vi "Keithley2200series_2_ST.vi"() -> ()   [LabVIEW 2010]
uses:
  <vilib>/Utility/error.llb/whitespace.ctl
  C:/Users/rad/Desktop/Keithley 2200 Series Power Supplies Ver 1.2 (LV2009)/Keithley 2200 Series/Keithley 2200 Series.lvlib
panel:
  in  "ИС":string="5962-9683901MPA"
  in  "№ ИС":string
  out "SEE1 Count 2":dbl
  out "SEE1 Count":dbl
  in  "SEE th 2":dbl
  in  "SEE th 1":dbl
  in  "+ИП2":bool
  out "MEAS 2":string
  in  "Cml set 2":dbl
  in  "Function(0:Voltage) 3":u16(ring) items=["Voltage", "Current"]
  in  "Out set 2":dbl
  in  "VISA resource name 2":refnum<visa-resource-name>
  in  "Cml set":dbl
  in  "Function(0:Voltage) 2":u16(ring) items=["Voltage", "Current"]
  in  "Out set":dbl
  in  "Файл записи замеров":path
  out "MEAS":string
  in  "VISA resource name":refnum<visa-resource-name>
  in  "stop":bool
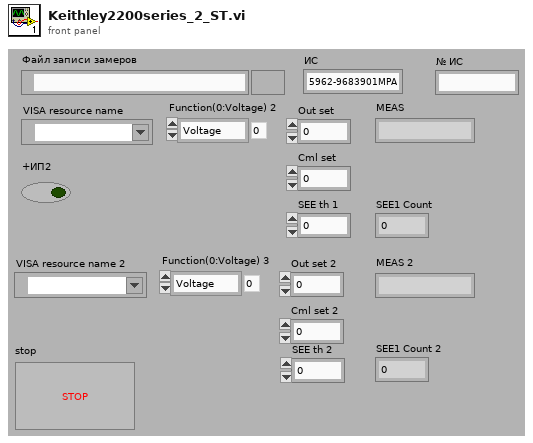
[diagram p1: front panel]
types:
  T1 = typedef "whitespace.ctl" = u16
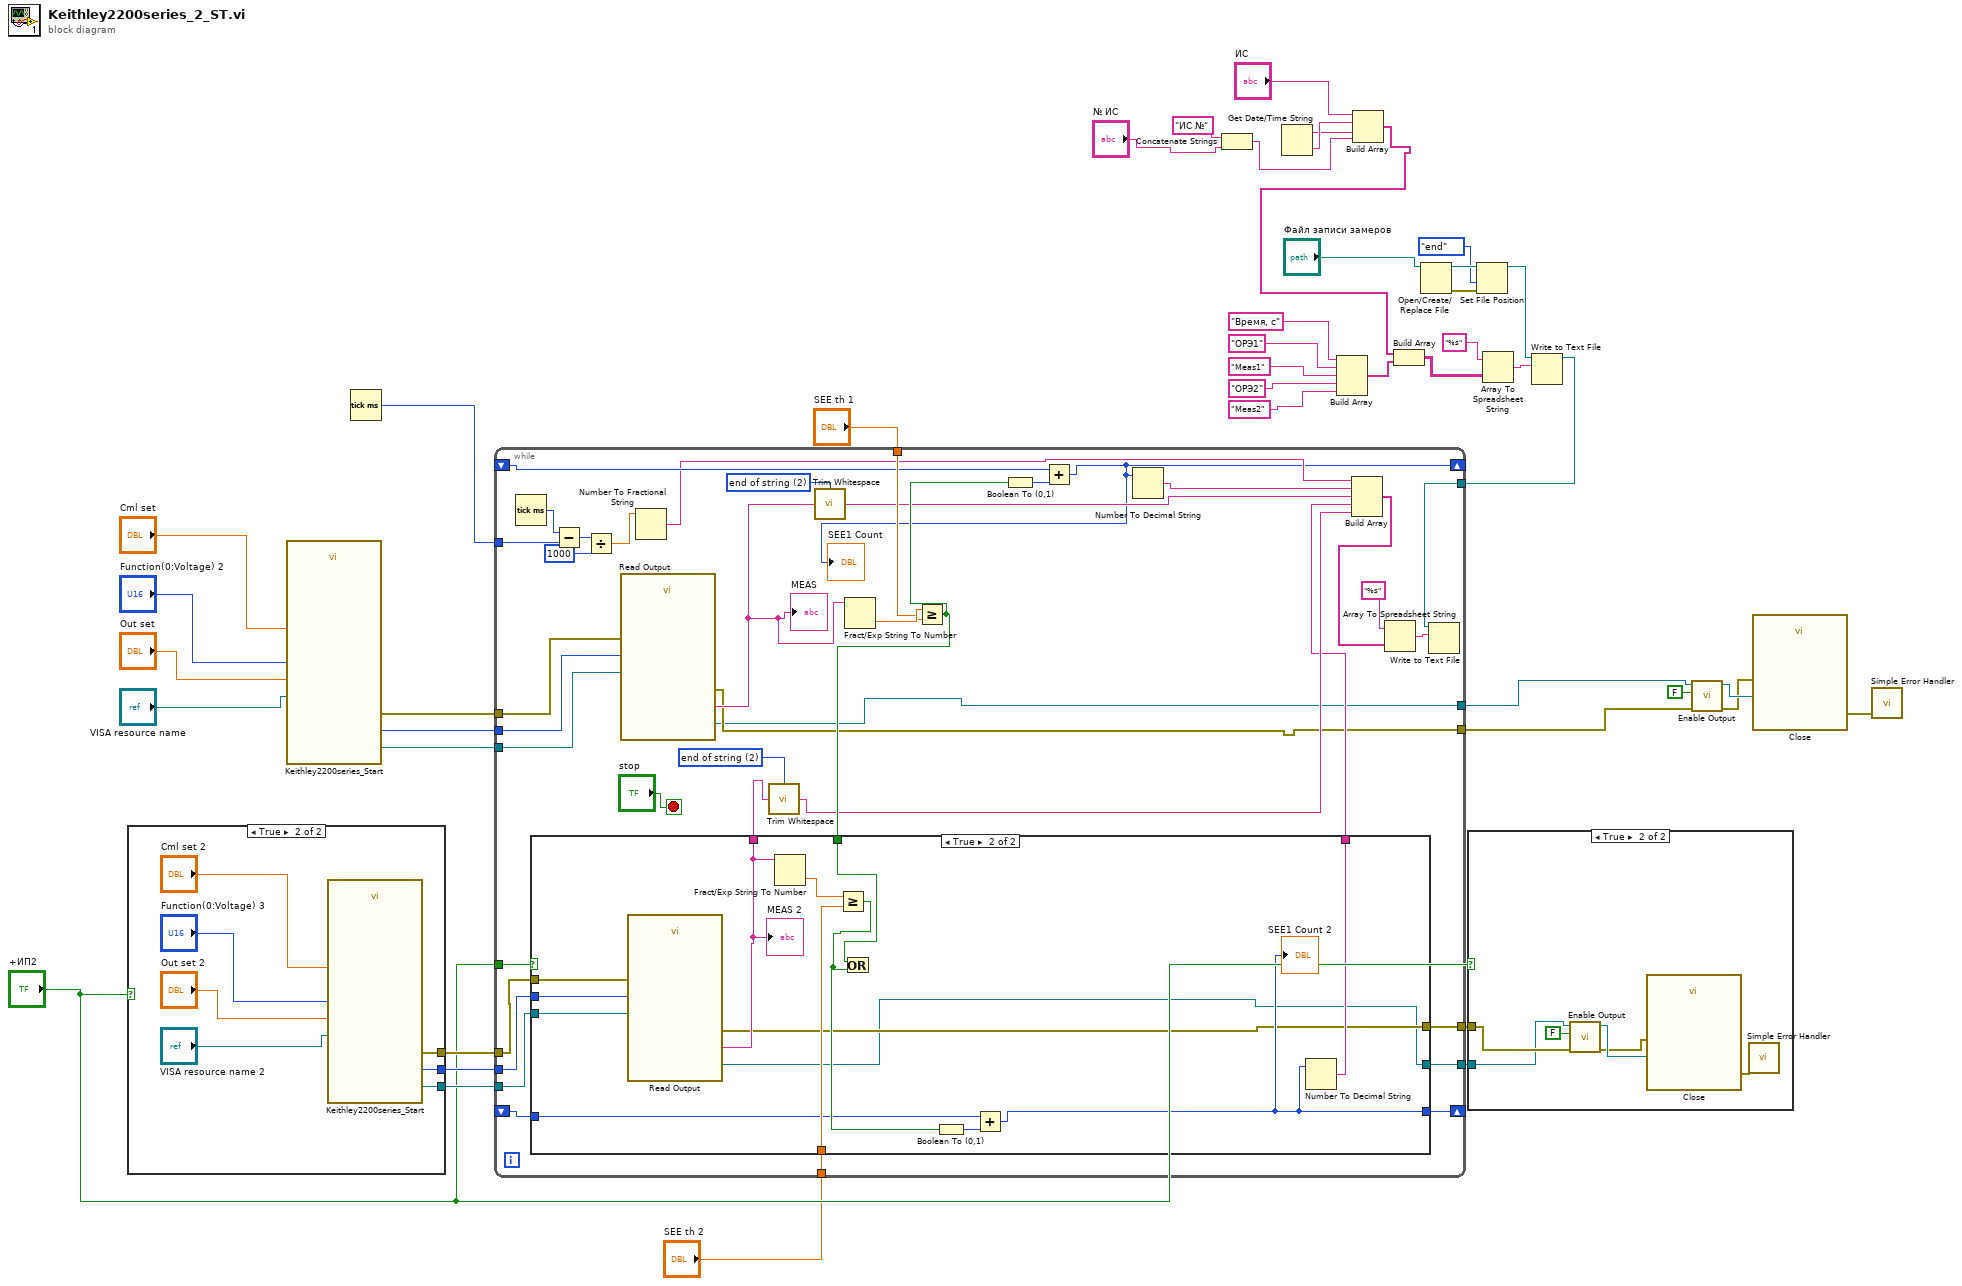
[diagram p0: block diagram]
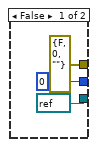
[diagram p3: hidden frame]
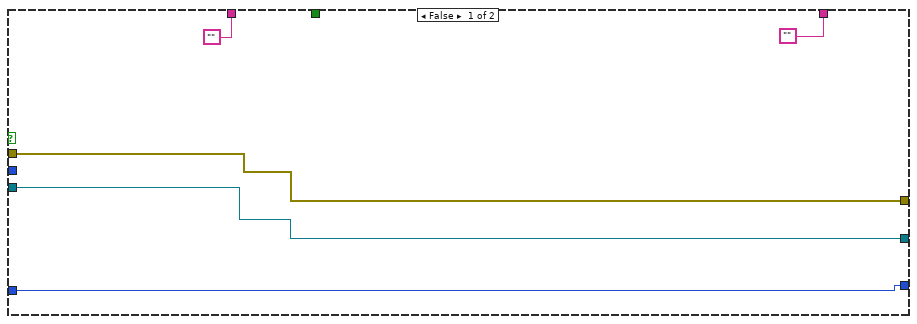
[diagram p4: hidden frame]
diagram:
  n1 = case shown="True" "+ИП2" {
    tunnel: [errorcluster {"status"=FALSE, "code"=0, "source"=""} ("error out 2") w50] -> w33
    tunnel: [0 ("Meas Func") w49] -> w32
    tunnel: [refnum<visa-resource-name> refnum ("VISA out") w48] -> w31
    frame False {
    }
    frame True {
      n2 = call "Keithley2200series_Start.vi"("VISA resource name 2"="VISA resource name 2", "Function(0:Voltage) 3"="Function(0:Voltage) 3", "Out set 2"="Out set 2", "Cml set 2"="Cml set 2") -> ("VISA out"=w48:refnum<visa-resource-name>, "Meas Func"=w49:i32, "error out 2"=w50:errorcluster)  [unwired: 1 in]
    }
  }
  n3 = call "Keithley2200series_Start.vi"("VISA resource name 2"="VISA resource name", "Function(0:Voltage) 3"="Function(0:Voltage) 2", "Out set 2"="Out set", "Cml set 2"="Cml set") -> ("VISA out"=w39:refnum<visa-resource-name>, "Meas Func"=w38:i32, "error out 2"=w37:errorcluster)  [unwired: 1 in]
  n4 = Tick Count (ms)() -> (millisecond timer value=w44:u32)
  n5 = Concatenate Strings("ИС №" ("string"), "№ ИС") -> (w5:string)
  n6 = Get Date/Time String() -> (date string=w8:string, time string=w9:string)  [unwired: 3 in]
  n7 = Build Array("Время, с", "ОРЭ1", "Meas1", "ОРЭ2", "Meas2") -> (w2:string[])
  n8 = Build Array("ИС", w9, w8, w5) -> (w1:string[])
  n9 = Build Array(w1, w2) -> (w3:string[][])
  n10 = Open/Create/Replace File(file path (use dialog)="Файл записи замеров") -> (refnum out=w13:refnum<file>, error out=w14:errorcluster)  [unwired: 5 in, 1 out]
  n11 = Set File Position(refnum=w13, from (0:start)=enum16{"start", "end", "current"}."end", error in=w14) -> (refnum out=w12:refnum<file>)  [unwired: 1 in, 1 out]
  n12 = Array To Spreadsheet String(array=w3, 3:"%s" ("format string")) -> (spreadsheet string=w17:string)  [unwired: 1 in]
  n13 = Write to Text File(file (use dialog)=w12, text=w17) -> (refnum out=w15:refnum<file>)  [unwired: 2 in, 2 out]
  n14 = while {
    tunnel: w44 -> [w92]
    tunnel: w39 -> [w88]
    tunnel: w38 -> [w87]
    tunnel: w37 -> [w86]
    tunnel: [w84] -> w35
    tunnel: [w83] -> w34
    tunnel: w33 -> [w82]
    tunnel: w32 -> [w81]
    tunnel: w31 -> [w80]
    tunnel: "+ИП2" -> [w79]
    tunnel: "SEE th 1" -> [w77]
    tunnel: "SEE th 2" -> [w76]
    tunnel: [w55] -> w24
    tunnel: [w56] -> w23
    shift-right: [w57] -> _
    shift-left: _ -> [w74]
    shift-right: [w71] -> _
    shift-left: _ -> [w72]
    tunnel: w15 -> [w68]
    stop <- "stop" stop-if-true
    w60 = T1 2 items=["both", "start of string", "end of string"] ("location (both)")
    w63 = T1 2 items=["both", "start of string", "end of string"] ("location (both)")
    n15 = Tick Count (ms)() -> (millisecond timer value=w93:u32)
    n16 = Subtract(x=w93, y=w92) -> (x-y=w91:u32)
    n17 = Divide(x=w91, y=u32 1000) -> (x/y=w89:dbl)
    n18 = call "Read Output.vi"("VISA resource name"=w88, "Measurement Function (0:Voltage)"=w87, "error in (no error)"=w86) -> ("VISA resource name out"=w55:refnum<visa-resource-name>, "Measurement"=w62:string, "error out"=w56:errorcluster)  [unwired: 10 in]
    "MEAS" <- w62
    n19 = Number To Fractional String(number=w89) -> (F-format string=w67:string)  [unwired: 3 in]
    n20 = call <vilib>:"Trim Whitespace.vi"("string"=w62, "location (both)"=w60) -> ("trimmed string"=w61:string)
    n21 = Fract/Exp String To Number(string=w62) -> (number=w78:dbl)  [unwired: 3 in, 1 out]
    n22 = Greater Or Equal?(x=w78, y=w77) -> (x >= y?=w73:bool)
    n23 = case shown="True" w79 {
      tunnel: [w98 w100] -> w84
      tunnel: [w97 w99] -> w83
      tunnel: ["" w109] -> w64
      tunnel: w82 -> [w98 w112]
      tunnel: w81 -> [_ w111]
      tunnel: w80 -> [w97 w110]
      tunnel: w76 -> [_ w108]
      tunnel: w73 -> [_ w106]
      tunnel: w72 -> [w96 w103]
      tunnel: [w96 w101] -> w71
      tunnel: ["" w102] -> w58
      frame False {
      }
      frame True {
        n24 = call "Read Output.vi"("VISA resource name"=w110, "Measurement Function (0:Voltage)"=w111, "error in (no error)"=w112) -> ("VISA resource name out"=w99:refnum<visa-resource-name>, "Measurement"=w109:string, "error out"=w100:errorcluster)  [unwired: 10 in]
        "MEAS 2" <- w109
        n25 = Fract/Exp String To Number(string=w109) -> (number=w107:dbl)  [unwired: 3 in, 1 out]
        n26 = Greater Or Equal?(x=w107, y=w108) -> (x >= y?=w104:bool)
        n27 = Or(x=w106, y=w104) -> ()  [unwired: 1 out]
        n28 = Boolean To (0,1)(Boolean=w104) -> (0, 1=w105:i16)
        n29 = Add(x=w103, y=w105) -> (x+y=w101:i16)
        "SEE1 Count 2" <- w101
        n30 = Number To Decimal String(number=w101) -> (decimal integer string=w102:string)  [unwired: 1 in]
      }
    }
    n31 = call <vilib>:"Trim Whitespace.vi"("string"=w64, "location (both)"=w63) -> ("trimmed string"=w59:string)
    n32 = Boolean To (0,1)(Boolean=w73) -> (0, 1=w75:i16)
    n33 = Add(x=w74, y=w75) -> (x+y=w57:i16)
    "SEE1 Count" <- w57
    n34 = Number To Decimal String(number=w57) -> (decimal integer string=w66:string)  [unwired: 1 in]
    n35 = Build Array(w67, w66, w61, w58, w59) -> (w65:string[])
    n36 = Array To Spreadsheet String(array=w65, 3:"%s" ("format string")) -> (spreadsheet string=w69:string)  [unwired: 1 in]
    n37 = Write to Text File(file (use dialog)=w68, text=w69) -> ()  [unwired: 2 in, 3 out]
  }
  n38 = case shown="True" "+ИП2" {
    tunnel: w35 -> [_ w116]
    tunnel: w34 -> [_ w115]
    frame False {
    }
    frame True {
      n39 = call "Enable Output.vi"("error in (no error)"=w116, "Enable Output (T: Enable)"=FALSE, "VISA resource name"=w115) -> ("error out"=w113:errorcluster, "VISA resource name out"=w114:refnum<visa-resource-name>)  [unwired: 7 in]
      n40 = call "Close.vi"("error in (no error)"=w113, "VISA resource name"=w114) -> ("error out"=w118:errorcluster)  [unwired: 9 in]
      n41 = call <vilib>:"Simple Error Handler.vi"("error in (no error)"=w118) -> ()  [unwired: 4 in, 5 out]
    }
  }
  n42 = call "Enable Output.vi"("error in (no error)"=w23, "Enable Output (T: Enable)"=FALSE, "VISA resource name"=w24) -> ("error out"=w28:errorcluster, "VISA resource name out"=w29:refnum<visa-resource-name>)  [unwired: 7 in]
  n43 = call "Close.vi"("error in (no error)"=w28, "VISA resource name"=w29) -> ("error out"=w36:errorcluster)  [unwired: 9 in]
  n44 = call <vilib>:"Simple Error Handler.vi"("error in (no error)"=w36) -> ()  [unwired: 4 in, 5 out]
